vi "Reverse Sort Test.vi"(8 "Error In":errorcluster) -> (0 "Error Out":errorcluster)   [LabVIEW 2023, in "Test.lvlib"]
uses:
  Test.lvlib
  <vilib>/addons/_JKI Toolkits/Caraya/classes/Assert/Assert Equal Value_Variant.vi
  <vilib>/addons/_JKI Toolkits/Caraya/classes/Test/Test.lvclass
  <vilib>/addons/_JKI Toolkits/Caraya/classes/Assert/Assert.lvclass
  File Path Operations/File and Path Operations.lvlib
panel:
  # "REVERSE ALPHABETICAL SORT TEST"
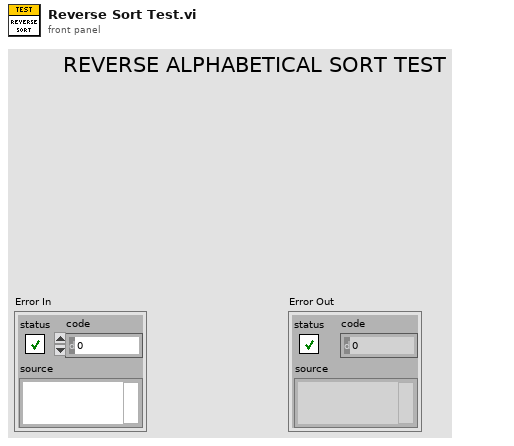
[diagram p1: front panel]
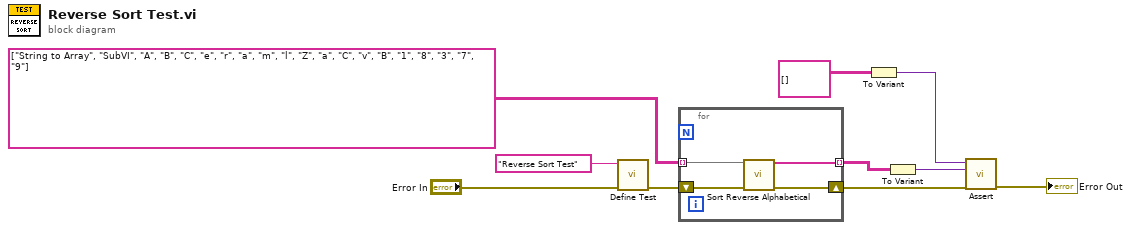
[diagram p0: block diagram]
diagram:
  n1 = call <vilib>:"Define Test.vi"("error in (no error)"="Error In", "Label (VI Title)"="Reverse Sort Test") -> ("error out"=w8:errorcluster)  [unwired: 8 in, 1 out]
  n2 = for {
    tunnel: string[][] [["String to Array", "SubVI", "A", "B", "C"], ["e", "r", "a", "m", "l"], ["Z", "a", "C", "v", "B"], ["1", "8", "3", "7", "9"]] -> [w12] mode=indexing
    shift-right: [w13] -> w7
    shift-left: w8 -> [w14]
    tunnel: [w11] -> w3 mode=indexing
    n3 = call "Sort Reverse Alphabetical.vi"("Unsorted Array"=w12, "Error In"=w14) -> ("Sorted Array"=w11:string[], "Error Out"=w13:errorcluster)  [unwired: 12 in]
  }
  n4 = To Variant(anything=string[][] [] ("Sorted Array")) -> (Variant=w1:variant)
  n5 = To Variant(anything=w3) -> (Variant=w4:variant)
  n6 = call-poly <vilib>:"Assert.vi"("error in (no error)"=w7, "Y"=w4, "X"=w1) -> ("error out"=→"Error Out":errorcluster)  [unwired: 7 in, 1 out]
